vi "build_commands.vi"(11 "T1_parameters":T1) -> (3 "instructions_array":T2(array[cluster]))   [LabVIEW 2018]
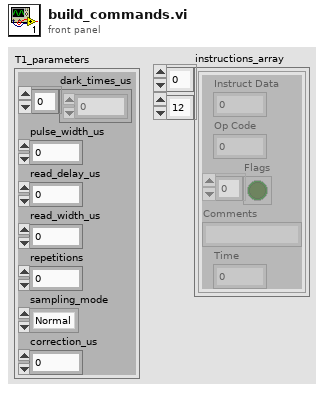
[diagram p1: front panel]
types:
  T1 = cluster{"dark_times_us":dbl[], "pulse_width_us":dbl, "read_delay_us":dbl, "read_width_us":dbl, "repetitions":i32, "sampling_mode":enum16{"Normal", "Sweep"}, "correction_us":dbl}
  T2 = cluster{"Instruct Data":i32, "Op Code":i32, "Flags":bool[], "Comments":string, "Time":dbl}[][]
  T3 = cluster{"Instruct Data":i32, "Op Code":i32, "Flags":bool[], "Comments":string, "Time":dbl}[]
  T4 = cluster{"Instruct Data":i32, "Op Code":i32, "Flags":bool[], "Comments":string, "Time":dbl}
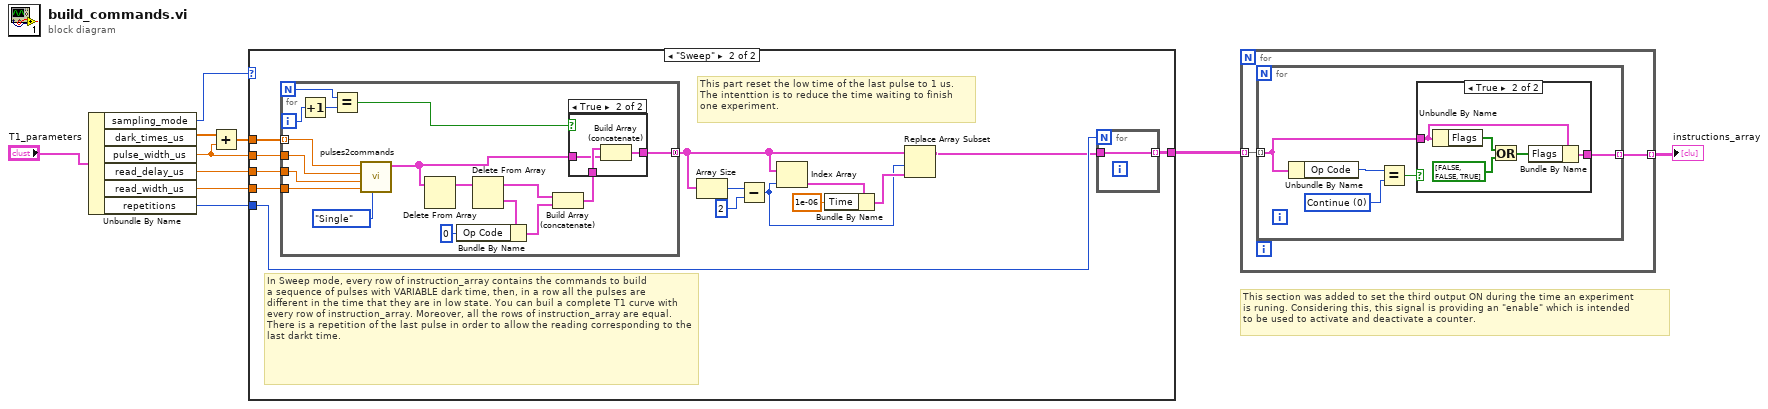
[diagram p0: block diagram]
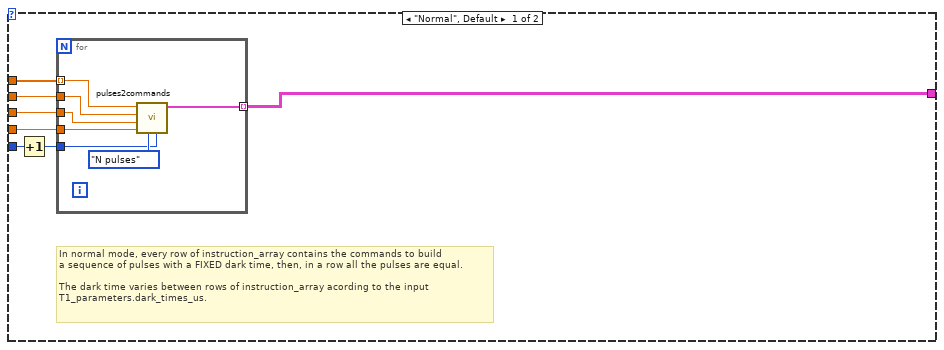
[diagram p3: hidden frame]
diagram:
  # "This section was added to set the third output ON during the time an experiment\nis runing. Considering this, this signal is providing an \"enable\" which is intended\nto be used to activate and deactivate a counter."
  n1 = Unbundle By Name("T1_parameters") -> ("sampling_mode"=w4:enum16{"Normal", "Sweep"}, "dark_times_us"=w5:dbl[], "pulse_width_us"=w7:dbl, "read_delay_us"=w8:dbl, "read_width_us"=w9:dbl, "repetitions"=w10:i32)
  n2 = Add(x=w5, y=w7) -> (x+y=w6:dbl[])
  n3 = case shown="\"Sweep\"" w4 {
    tunnel: w6 -> [w13 w38]
    tunnel: w7 -> [w14 w37]
    tunnel: w8 -> [w15 w36]
    tunnel: w9 -> [w16 w35]
    tunnel: w10 -> [w17 w34]
    tunnel: [w11 w33] -> w2
    frame "Normal", Default {
      # "In normal mode, every row of instruction_array contains the commands to build \na sequence of pulses with a FIXED dark time, then, in a row all the pulses are equal.\n\nThe dark time varies between rows of instruction_array acording to the input\nT1_parameters.dark_times_us."
      n4 = Increment(x=w17) -> (x+1=w12:i32)
      n5 = for {
        tunnel: w12 -> [w23]
        tunnel: w16 -> [w22]
        tunnel: w15 -> [w21]
        tunnel: w14 -> [w20]
        tunnel: w13 -> [w19] mode=indexing
        tunnel: [w18] -> w11 mode=indexing
        n6 = call "pulses2commands.vi"("N_pulses"=w23, "running_mode"=enum16{"Continuous", "Single", "N pulses"}."N pulses", "read_width_us"=w22, "read_delay_us"=w21, "pulse_width_us"=w20, "pulse_period_us"=w19) -> ("instructions_array"=w18:T3)  [unwired: 4 in, 1 out]
      }
    }
    frame "Sweep" {
      # "This part reset the low time of the last pulse to 1 us.\nThe intenttion is to reduce the time waiting to finish\none experiment."
      # "In Sweep mode, every row of instruction_array contains the commands to build \na sequence of pulses with VARIABLE dark time, then, in a row all the pulses are \ndifferent in the time that they are in low state. You can buil a complete T1 curve with every row of instruction_array. Moreover, all the rows of instruction_array are equal.\nThere is a repetition of the last pulse in order to allow the reading corresponding to the last darkt time."
      n7 = for {
        N -> [w49]
        tunnel: w38 -> [w56] mode=indexing
        tunnel: w37 -> [w55]
        tunnel: w36 -> [w54]
        tunnel: w35 -> [w53]
        tunnel: [w40] -> w28 mode=concatenating
        i -> [w51]
        n8 = Increment(x=w51) -> (x+1=w50:i32)
        n9 = Equal?(x=w49, y=w50) -> (x = y?=w43:bool)
        n10 = call "pulses2commands.vi"("running_mode"=enum16{"Continuous", "Single", "N pulses"}."Single", "read_width_us"=w53, "read_delay_us"=w54, "pulse_width_us"=w55, "pulse_period_us"=w56) -> ("instructions_array"=w41:T3)  [unwired: 5 in, 1 out]
        n11 = Delete From Array(array=w41) -> (array with subset deleted=w46:T3)  [unwired: 2 in, 1 out]
        n12 = Delete From Array(array=w46) -> (deleted portion=w45:T4, array with subset deleted=w44:T3)  [unwired: 2 in]
        n13 = Bundle By Name(cluster=w45, "Op Code"=0) -> (w47:T4)
        n14 = Build Array (concatenate)(w44, w47) -> (w42:T3)
        n15 = case shown="True" w43 {
          tunnel: w42 -> [w57 w60]
          tunnel: [w57 w59] -> w40
          tunnel: w41 -> [_ w58]
          frame False {
          }
          frame True {
            n16 = Build Array (concatenate)(w60, w58) -> (w59:T3)
          }
        }
      }
      n17 = Array Size(array=w28) -> (size(s)=w32:i32)
      n18 = Subtract(x=w32, y=2) -> (x-y=w26:i32)
      n19 = Index Array(array=w28, index=w26) -> (element=w30:T4)
      n20 = Bundle By Name(cluster=w30, "Time"=1e-06) -> (w27:T4)
      n21 = Replace Array Subset(array=w28, new element=w27, index=w26) -> (w25:T3)
      n22 = for {
        N: w34 -> [_]
        tunnel: w25 -> [w39]
        tunnel: [w39] -> w33 mode=indexing
      }
    }
  }
  n23 = for {
    tunnel: w2 -> [w62] mode=indexing
    tunnel: [w61] -> w1 mode=indexing
    n24 = for {
      tunnel: w62 -> [w64] mode=indexing
      tunnel: [w63] -> w61 mode=indexing
      w66 = 0 items=["Continue", "Stop", "Loop", "End Loop", "JSR", "RTS", "Branch", "Long Delay", "Wait"] ("Op Code")
      n25 = Unbundle By Name(w64) -> ("Op Code"=w67:i32)
      n26 = Equal?(x=w67, y=w66) -> (x = y?=w65:bool)
      n27 = case shown="True" w65 {
        tunnel: w64 -> [w68 w71]
        tunnel: [w68 w69] -> w63
        frame False {
        }
        frame True {
          n28 = Unbundle By Name(w71) -> ("Flags"=w73:bool[])
          n29 = Or(x=w73, y=bool[] [FALSE, FALSE, TRUE] ("Flags")) -> (x .or. y?=w70:bool[])
          n30 = Bundle By Name(cluster=w71, "Flags"=w70) -> (w69:T4)
        }
      }
    }
  }
  "instructions_array" <- w1
